vi "ZScan-J2 .vi"() -> ()   [LabVIEW 2014]
uses:
  <vilib>/Analysis/NI_AALBase.lvlib
panel:
  out "size(s)":i32
  out "Histogram Graph":T1(graph)
  out "median":dbl format="%0.4f"
  out "variance fechada":dbl format="%4f"
  out "standard deviation fechada":dbl format="%4f"
  out "mean fechada":dbl format="%4f"
  out "variance aberta":dbl format="%4f"
  out "standard deviation aberta":dbl format="%4f"
  out "mean aberta":dbl format="%4f"
  out "Process time":string="0:00:50"
  out "Waveform Graph 3":dbl[][](graph)
  out "subarray 2":dbl[](array[numeric])
  out "subarray":dbl[](array[numeric])
  out "tf":dbl
  out "ti":dbl
  out "tf":dbl
  out "ti":dbl
  out "Waveform Graph 2":dbl[](graph)
  out "Waveform Graph":dbl[](graph)
  out "?":dynamicdata(graph)=[{"t0"=timestamp(3608319334.616045 s since 1904-01-01), "dt"=9.999999999999972e-06, "Y"=array[2000 elements], "attributes"=variant("NI_ChannelName"=variant(string "fenda_fech (Trigger)"), "NI_OriginalChannelName"=variant(string "fenda_fech"), "NI_UnitDescription"=variant(string "Volts"))}, {"t0"=timestamp(3608319334.6160502 s since 1904-01-01), "dt"=9.999999999999972e-06, "Y"=array[2000 elements], "attributes"=variant("NI_ChannelName"=variant(string "fenda_abert (Trigger)"), "NI_OriginalChannelName"=variant(string "fenda_abert"), "NI_UnitDescription"=variant(string "Volts"))}]
  out "Fenda Aberta":cluster{"Y":dbl[], "Y":dbl[]}[](graph)=[{"Y"=[0.0, 0.05, 0.1, 0.15000000000000002, 0.2, 0.25, 0.30000000000000004, 0.35000000000000003, 0.4, 0.45, 0.5, 0.55, 0.6000000000000001, 0.65, 0.7000000000000001, 0.75, 0.8, 0.8500000000000001, 0.9, 0.9500000000000001, 1.0, 1.05, 1.1, 1.1500000000000001, 1.2000000000000002, 1.25, 1.3, 1.35, 1.4000000000000001, 1.4500000000000002, 1.5, 1.55, 1.6, 1.6500000000000001, 1.7000000000000002, 1.75, 1.8, 1.85, 1.9000000000000001, 1.9500000000000002, 2.0, 2.0500000000000003, 2.1, 2.15, 2.2, 2.25, 2.3000000000000003, 2.35, 2.4000000000000004, 2.45, 2.5, 2.5500000000000003, 2.6, 2.6500000000000004, 2.7, 2.75, 2.8000000000000003, 2.85, 2.9000000000000004, 2.95, 3.0], "Y"=[1.0003560119658135, 1.0012013375370006, 1.0011098447584892, 1.0003868333205452, 1.0005911311098947, 1.00176519837504, 1.0016057017995816, 1.0010135652990357, 1.0000765053622271, 0.9994335285770138, 0.999866472092084, 1.0013086578544201, 0.9983210531853085, 1.0013003326270395, 0.9987277013791608, 0.9999850836921477, 1.0013154033205038, 1.0003449476028676, 1.00530783597501, 1.0039138176163034, 1.0020720153786586, 0.9974475595275478, 1.0025710719122825, 1.0004536737753678, 0.9971856721413305, 0.9991163463336346, 1.002352334676977, 0.9992227742532884, 1.0009590150136298, 1.0000404565927934, 1.0014055358415577, 1.003866651633942, 1.0011576095643933, 1.0009409138118541, 1.001613479435038, 1.0000868071678926, 1.0016518693754177, 1.000614985100232, 1.0009343420915624, 1.000727082698536, 1.0013886849015161, 1.0010159171435018, 0.9999366457422144, 0.9993990398035298, 1.001219758706698, 1.0001163511824618, 1.00322890499305, 1.000332245507808, 0.9993934380432397, 1.00042841763974, 1.0013901823583342, 1.0006026083888238, 1.0015125224155137, 1.0016120200132204, 1.0013346501890377, 1.0006682992031124, 1.0002607058936361, 0.9995807130678198, 1.0007896268833816, 0.9988210755118042, 1.0011170211549907]}]
  out "Numeric":i32=399
  out "divisão":dbl=1.0004767592065456
  out "?":cluster{"Y":dbl[], "Y":dbl[]}[](graph)=[{"Y"=[0.0, 0.05, 0.1, 0.15000000000000002, 0.2, 0.25, 0.30000000000000004, 0.35000000000000003, 0.4, 0.45, 0.5, 0.55, 0.6000000000000001, 0.65, 0.7000000000000001, 0.75, 0.8, 0.8500000000000001, 0.9, 0.9500000000000001, 1.0, 1.05, 1.1, 1.1500000000000001, 1.2000000000000002, 1.25, 1.3, 1.35, 1.4000000000000001, 1.4500000000000002, 1.5, 1.55, 1.6, 1.6500000000000001, 1.7000000000000002, 1.75, 1.8, 1.85, 1.9000000000000001, 1.9500000000000002, 2.0, 2.0500000000000003, 2.1, 2.15, 2.2, 2.25, 2.3000000000000003, 2.35, 2.4000000000000004, 2.45, 2.5, 2.5500000000000003, 2.6, 2.6500000000000004, 2.7, 2.75, 2.8000000000000003, 2.85, 2.9000000000000004, 2.95, 3.0], "Y"=[0.9946653153115961, 0.9935440305988315, 0.9923499742414911, 0.9937057682962681, 0.9928758206473707, 0.99272134080173, 0.9920005276901647, 0.991928489834513, 0.9902859622147167, 0.9893941409964322, 0.9881312874958551, 0.9885748328409064, 0.9879498665044865, 0.9854119919449715, 0.9852206725828448, 0.9836834880850088, 0.9835336656068788, 0.9827510235849405, 0.9800567220741527, 0.9790354014607947, 0.9757861932090093, 0.9736287121932531, 0.9733110209958593, 0.9672187803332435, 0.9698255374557961, 0.9657078625477571, 0.9626698627703867, 0.959377701265833, 0.9597152236942302, 0.9587367649583391, 0.9695734847735785, 0.9820871170728013, 1.002228084693104, 1.021092956837102, 1.0358424149299008, 1.0425541650858727, 1.0444607271332977, 1.0425264734021085, 1.040303254766623, 1.0356485771759765, 1.0342601383048378, 1.029567545315073, 1.025784158272743, 1.0194392035719846, 1.0170617096384111, 1.0163238004274322, 1.0148377255880559, 1.0106373325058826, 1.0105773205187942, 1.0082170620349111, 1.00734634006814, 1.0053797911693145, 1.0053318513574079, 1.004546640720759, 1.0031843858366258, 1.0022071728600348, 1.0044572995782834, 1.002016970955132, 1.0003831738069051, 1.0034770905857964, 1.0004767592065456]}]
  out "transmitancia aberta":dbl=1.0011170211549907
  out "voltagem final aberta":dbl=0.907696895189052
  out "voltagem inicial aberta":dbl=0.9066841098574473
  in  "taxa":dbl=75000.0
  out "já realizadas":i32=60
  out "transmitancia fechada":dbl=1.0015943129116558
  out "voltagem final fechada":dbl=1.0322824425424475
  out "voltagem inicial fechada":dbl=1.0306392810294427
  in  "tempo final":dbl=0.0048
  in  "tempo inicial":dbl=2.5e-05
  in  "número de pontos":i32=60
  in  "número de médias":i32=400
  out "?":dynamicdata(graph)=[{"t0"=timestamp(3608319334.616045 s since 1904-01-01), "dt"=9.999999999999972e-06, "Y"=array[2000 elements], "attributes"=variant("NI_ChannelName"=variant(string "fenda_fech (Trigger)"), "NI_OriginalChannelName"=variant(string "fenda_fech"), "NI_UnitDescription"=variant(string "Volts"))}, {"t0"=timestamp(3608319334.6160502 s since 1904-01-01), "dt"=9.999999999999972e-06, "Y"=array[2000 elements], "attributes"=variant("NI_ChannelName"=variant(string "fenda_abert (Trigger)"), "NI_OriginalChannelName"=variant(string "fenda_abert"), "NI_UnitDescription"=variant(string "Volts"))}]
  in  "Distância motor passo por ciclo (cm)":dbl=0.05
  in  "Sentido":bool[](array[boolean])=[FALSE, FALSE]
  # "S=?\nP0=?"
  # "A taxa do carro atual é 44642,43845."
  # "OBS: Ajustar a taxa nas constantes no diagrama de bloco e a frequência no painel frontal para 10,3Hz."
  # "Motor Passo"
  # "Direção do carrinho:"
  # "<----"
  # "---->"
  # "Fenda fechada = AI0\nFenda aberta = AI2"
  # "Osciloscópio"
  # "Z-Scan"
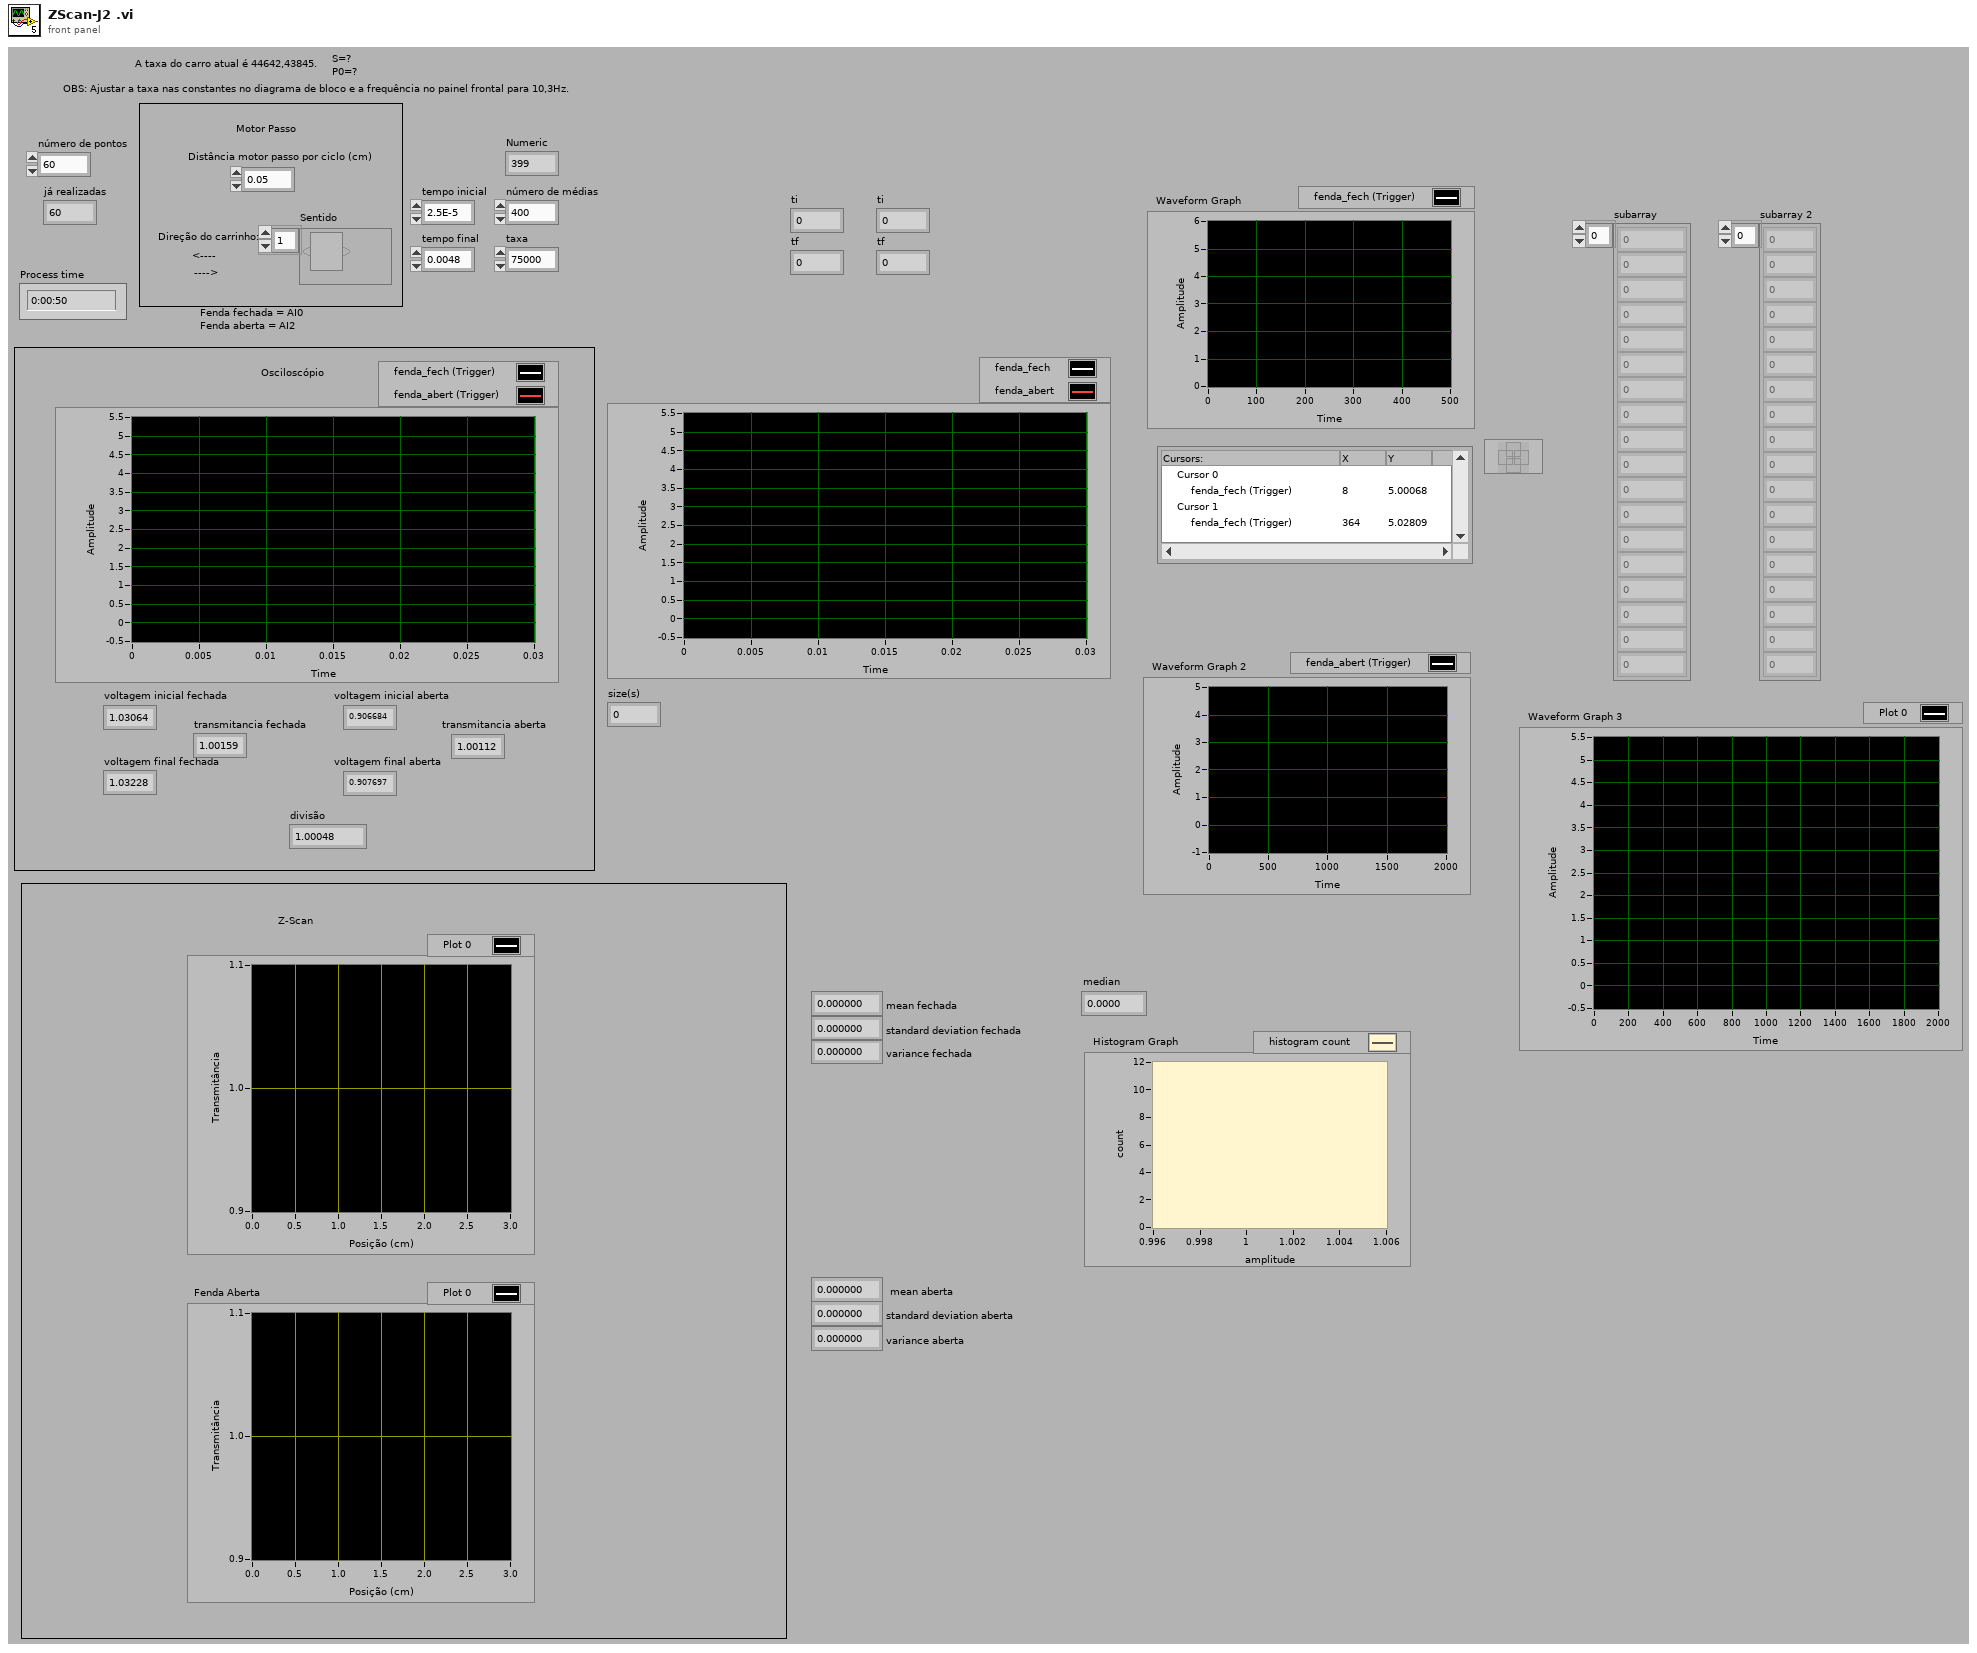
[diagram p1: front panel]
types:
  T1 = cluster{"X Values":dbl[], "Histogram: h(x)":i32[]}
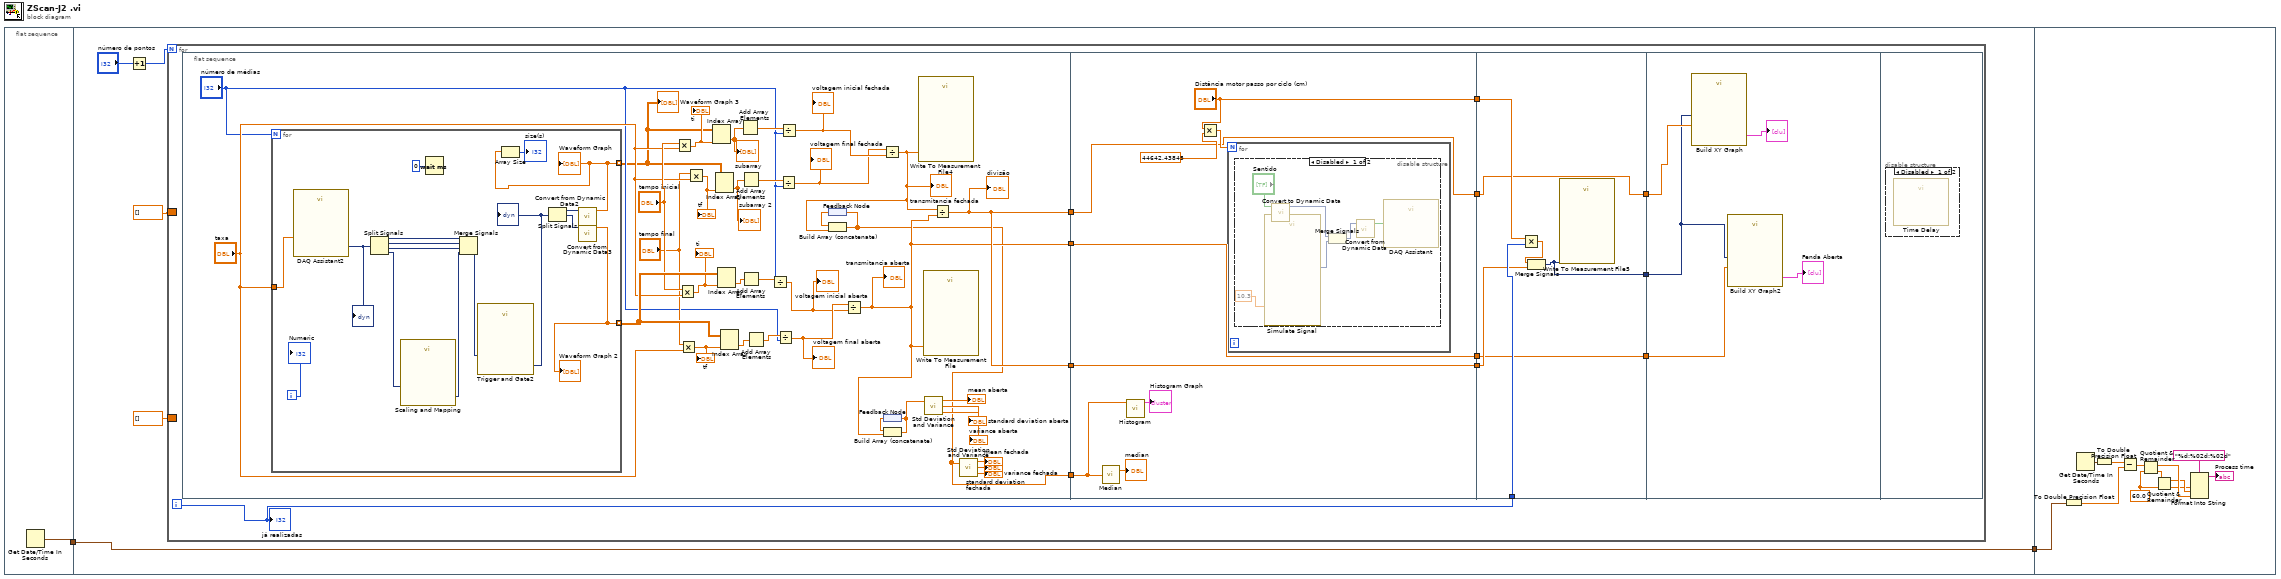
[diagram p0: block diagram]
diagram:
  n1 = flat-sequence {
    tunnel: [w3] -> w2
    tunnel: w2 -> [w6]
    tunnel: [w6] -> w1
    tunnel: w1 -> [w109]
    frame #0 {
      n2 = Get Date/Time In Seconds() -> (seconds since 1Jan1904=w3:timestamp)
    }
    frame #1 {
      n3 = Increment(x="número de pontos") -> (x+1=w8:i32)
      n4 = for {
        N: w8 -> [_]
        border: dbl[] [] -> [_]
        border: dbl[] [] -> [_]
        i -> [w20]
        n5 = flat-sequence {
          tunnel: [w35] -> w17
          tunnel: [w29] -> w13
          tunnel: [w35] -> w10
          tunnel: [w21] -> w9
          tunnel: ["Distância motor passo por ciclo (cm)"] -> w19
          tunnel: [w77] -> w18
          tunnel: w17 -> [w77]
          tunnel: [w76] -> w14
          tunnel: w13 -> [w76]
          tunnel: [w75] -> w11
          tunnel: w10 -> [w75]
          tunnel: w9 -> [w73]
          tunnel: w20 -> [w92]
          tunnel: w19 -> [w89]
          tunnel: w18 -> [w91]
          tunnel: [w90] -> w16
          tunnel: [w88] -> w15
          tunnel: w14 -> [w88]
          tunnel: [w87] -> w12
          tunnel: w11 -> [w87]
          tunnel: w16 -> [w94]
          tunnel: w15 -> [w96]
          tunnel: w12 -> [w95]
          frame #0 {
            n6 = for {
              N: "número de médias" -> [_]
              tunnel: "taxa" -> [w70]
              tunnel: [w57] -> w33 mode=indexing
              tunnel: [w59] -> w49 mode=indexing
              i -> [w71]
              n7 = call "DAQ Assistant2"("rate"=w70) -> ("data"=w63:dynamicdata)  [unwired: 16 in, 2 out]
              "?" <- w63
              n8 = Split Signals(w63) -> (w67:dynamicdata, w69:dynamicdata, w68:dynamicdata, w64:dynamicdata)  [unwired: 4 in]
              n9 = call "Scaling and Mapping"("Signals"=w64) -> ("Scaled Signals"=w62:dynamicdata)  [unwired: 9 in, 1 out]
              n10 = Wait (ms)(milliseconds to wait=u32 0) -> ()  [unwired: 1 out]
              n11 = Merge Signals(w67, w69, w68, w62) -> (w66:dynamicdata)
              n12 = call "Trigger and Gate2"("Signals"=w66) -> ("Triggered Signals"=w65:dynamicdata)  [unwired: 7 in, 3 out]
              "?" <- w65
              n13 = Split Signals(w65) -> (w61:dynamicdata, w60:dynamicdata)  [unwired: 3 in, 1 out]
              n14 = call "Convert from Dynamic Data2"("Dynamic Data Type"=w61) -> ("Array"=w57:dbl[])  [unwired: 3 in]
              "Waveform Graph" <- w57
              n15 = Array Size(array=w57) -> (size(s)=→"size(s)":i32)
              n16 = call "Convert from Dynamic Data3"("Dynamic Data Type"=w60) -> ("Array"=w59:dbl[])  [unwired: 3 in]
              "Waveform Graph 2" <- w59
              "Numeric" <- w71
            }
            "Waveform Graph 3" <- w33
            n17 = Multiply(x="tempo inicial", y="taxa") -> (x*y=w53:dbl)
            "ti" <- w53
            n18 = Multiply(x="tempo inicial", y="taxa") -> (x*y=w48:dbl)
            "ti" <- w48
            n19 = Multiply(x="tempo final", y="taxa") -> (x*y=w47:dbl)
            "tf" <- w47
            n20 = Multiply(x="tempo final", y="taxa") -> (x*y=w51:dbl)
            "tf" <- w51
            n21 = Index Array(array=w33, index (col)=w53) -> (element=w40:dbl[])  [unwired: 1 in]
            "subarray" <- w40
            n22 = Index Array(array=w33, index (col)=w51) -> (element=w50:dbl[])  [unwired: 1 in]
            "subarray 2" <- w50
            n23 = Index Array(array=w49, index (col)=w48) -> (element=w46:dbl[])  [unwired: 1 in]
            n24 = Index Array(array=w49, index (col)=w47) -> (element=w45:dbl[])  [unwired: 1 in]
            n25 = Add Array Elements(numeric array=w40) -> (sum=w54:dbl)
            n26 = Add Array Elements(numeric array=w50) -> (sum=w55:dbl)
            n27 = Add Array Elements(numeric array=w46) -> (sum=w44:dbl)
            n28 = Add Array Elements(numeric array=w45) -> (sum=w43:dbl)
            n29 = Divide(x=w44, y="número de médias") -> (x/y=w41:dbl)
            "voltagem inicial aberta" <- w41
            n30 = Divide(x=w43, y="número de médias") -> (x/y=w42:dbl)
            "voltagem final aberta" <- w42
            n31 = Divide(x=w55, y="número de médias") -> (x/y=w34:dbl)
            "voltagem final fechada" <- w34
            n32 = Divide(x=w54, y="número de médias") -> (x/y=w52:dbl)
            "voltagem inicial fechada" <- w52
            n33 = feedback #1() -> (w32:dbl[])
            n34 = Divide(x=w42, y=w41) -> (x/y=w29:dbl)
            "transmitancia aberta" <- w29
            n35 = Divide(x=w34, y=w52) -> (x/y=w31:dbl)
            "transmitancia fechada" <- w31
            n36 = Build Array (concatenate)(w32, w31) -> (w21:dbl[])
            n37 = feedback-in #1(w21) -> ()
            n38 = feedback #2() -> (w30:dbl[])
            n39 = Build Array (concatenate)(w30, w29) -> (w28:dbl[])
            n40 = feedback-in #2(w28) -> ()
            n41 = call "Write To Measurement File4"("Signals"=w31) -> ()  [unwired: 16 in, 3 out]
            n42 = call "Write To Measurement File"("Signals"=w29) -> ()  [unwired: 16 in, 3 out]
            n43 = call <vilib>:"Std Deviation and Variance.vi"("X"=w28) -> ("mean"=→"mean aberta":dbl, "standard deviation"=→"standard deviation aberta":dbl, "variance"=→"variance aberta":dbl)  [unwired: 1 in]
            n44 = Divide(x=w31, y=w29) -> (x/y=w35:dbl)
            "divisão" <- w35
            n45 = call <vilib>:"Std Deviation and Variance.vi"("X"=w21) -> ("mean"=→"mean fechada":dbl, "standard deviation"=→"standard deviation fechada":dbl, "variance"=→"variance fechada":dbl)  [unwired: 1 in]
          }
          frame #1 {
            n46 = call <vilib>:"Median.vi"("X"=w73) -> ("median"=→"median":dbl)  [unwired: 1 out]
            n47 = call <vilib>:"Histogram.vi"("X"=w73) -> ("Histogram Graph"=→"Histogram Graph":T1)  [unwired: 7 in, 3 out]
            n48 = Multiply(x="Distância motor passo por ciclo (cm)", y=44642.43845) -> (x*y=w79:dbl)
            n49 = for {
              N: w79 -> [_]
              n50 = disable-structure shown="Disabled" {
                frame Disabled {
                  n51 = call "Simulate Signal"("Frequency"=10.3) -> ("Square"=w83:dynamicdata)  [unwired: 13 in, 1 out]
                  n52 = call "Convert to Dynamic Data"("Array"="Sentido") -> ("Dynamic Data Type"=w85:dynamicdata)  [unwired: 3 in]
                  n53 = Merge Signals(w85, w83) -> (w84:dynamicdata)
                  n54 = call "Convert from Dynamic Data"("Dynamic Data Type"=w84) -> ("Array"=w86:bool[])  [unwired: 3 in]
                  n55 = call "DAQ Assistant"("data"=w86) -> ()  [unwired: 17 in, 2 out]
                }
                frame Enabled {
                }
              }
            }
          }
          frame #2 {
            n56 = Multiply(x=w89, y=w92) -> (x*y=w93:dbl)
            n57 = Merge Signals(w93, w91) -> (w90:dynamicdata)
            n58 = call "Write To Measurement File5"("Signals"=w90) -> ()  [unwired: 16 in, 3 out]
          }
          frame #3 {
            n59 = call "Build XY Graph"("Y Input"=w95, "X Input"=w94) -> ("XY Graph"=→"?":cluster{"Y":dbl[], "Y":dbl[]}[])  [unwired: 8 in, 1 out]
            n60 = call "Build XY Graph2"("Y Input"=w96, "X Input"=w94) -> ("XY Graph"=→"Fenda Aberta":cluster{"Y":dbl[], "Y":dbl[]}[])  [unwired: 8 in, 1 out]
          }
          frame #4 {
            n61 = disable-structure shown="Disabled" {
              frame Disabled {
                n62 = call "Time Delay"() -> ()  [unwired: 11 in, 1 out]
              }
              frame Enabled {
              }
            }
          }
        }
        "já realizadas" <- w20
      }
    }
    frame #2 {
      w106 = 60.0 ("y")
      n63 = To Double Precision Float(number=w109) -> (double precision float=w110:dbl)
      n64 = Get Date/Time In Seconds() -> (seconds since 1Jan1904=w108:timestamp)
      n65 = To Double Precision Float(number=w108) -> (double precision float=w102:dbl)
      n66 = Subtract(x=w102, y=w110) -> (x-y=w101:dbl)
      n67 = Quotient & Remainder(x=w101, y=w106) -> (x-y*floor(x/y)=w105:dbl, floor(x/y)=w107:dbl)
      n68 = Quotient & Remainder(x=w107, y=w106) -> (x-y*floor(x/y)=w104:dbl, floor(x/y)=w103:dbl)
      n69 = Format Into String(format string="%d:%02d:%02d", w103, w104, w105) -> (resulting string=→"Process time":string)  [unwired: 2 in, 1 out]
    }
  }
